vi "CANopen Read SDO.vi"() -> ()   [LabVIEW 2016]
doc: "This example demonstrates how to read CANopen SDO from the device."
uses:
  <vilib>/userdefined/High Color/nirio_resource_hc.ctl
  <vilib>/FPGAPlugInAG/cRIO-9033/niLvFpga_Open_cRIO-9033.vi
  <vilib>/rvi/interface/common/dynamic/niFpgaDynamicAddResources.vi
  <vilib>/CANopenLib/CANOPEN.llb/CANopen Interface Create.vi
  <vilib>/CANopenLib/CANOPEN.llb/CANopen SDO Create.vi
  <vilib>/CANopenLib/CANOPEN.llb/CANopen SDO Read [STR].vi
  <vilib>/CANopenLib/CANOPEN.llb/CANopen SDO Close.vi
  <vilib>/CANopenLib/CANOPEN.llb/CANopen Interface Close.vi
  <vilib>/FPGAPlugInAG/Dynamic/niLvFpga_Close_Dynamic.vi
  <vilib>/rvi/interface/nirviOpenFPGA/nirviOpenFPGA.xnode
  Users/s163601/Desktop/05-28/FPGA Bitfiles/project_FPGATarget_MainFPGA_S9ZLErdeBuw.lvbitx
  Users/s163601/Desktop/05-28/RT/FPGA/MainFPGA.vi
  <vilib>/rvi/interface/nirviCloseFPGA/nirviCloseFPGA.xnode
panel:
  out "description":string
  in  "error in":errorcluster
  out "manufacturer device name":string
  out "completion code":u32 format="%.0x"
  in  "sub-index":u8 format="%.0x"
  in  "object index":u16=4104 format="%.0x"
  in  "node-ID":u8=1 min=1 max=127 step=1
  in  "baud rate":u32(ring)=2 items=["1 Mbit/s"=0, "800 kbit/s"=1, "500 kbit/s"=2, "250 kbit/s"=3, "125 kbit/s"=4, "50 kbit/s"=6, "20 kbit/s"=7, "10 kbit/s"=8]
  in  "CANopen interface":u32(ring) items=["CANopen01", "CANopen02", "CANopen03", "CANopen04", "CANopen05", "CANopen06", "CANopen07", "CANopen08", "CANopen09", "CANopen10", "CANopen11", "CANopen12", "CANopen13", "CANopen14", "CANopen15", "CANopen16", "CANopen17", "CANopen18", "CANopen19", "CANopen20", "CANopen21", "CANopen22", "CANopen23", "CANopen24", "CANopen25", "CANopen26", "CANopen27", "CANopen28", "CANopen29", "CANopen30", "CANopen31", "CANopen32"]
  # "Overview: This example demonstrates how to read CANopen SDO from the device.\nRequirements: Connect CANopen module with a slave device. \nInstructions:\n1. Specify the values of CANopen interface, baud rate of the CANopen interface and node-ID of the slave device.\n2. Run this VI."
  # "Create CANopen interface and SDO object"
  # "Read SDO data"
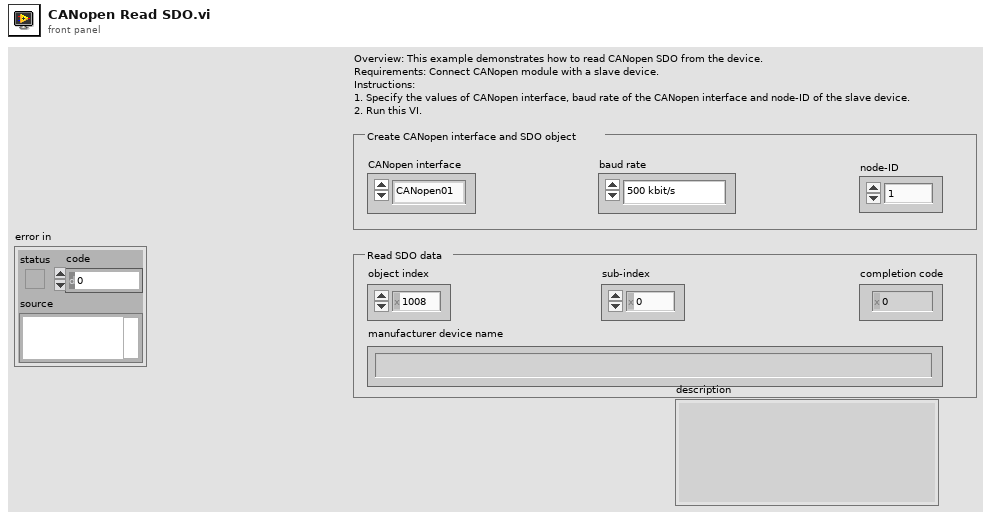
[diagram p1: front panel]
types:
  T1 = typedef "nirio_resource_hc.ctl" = tag
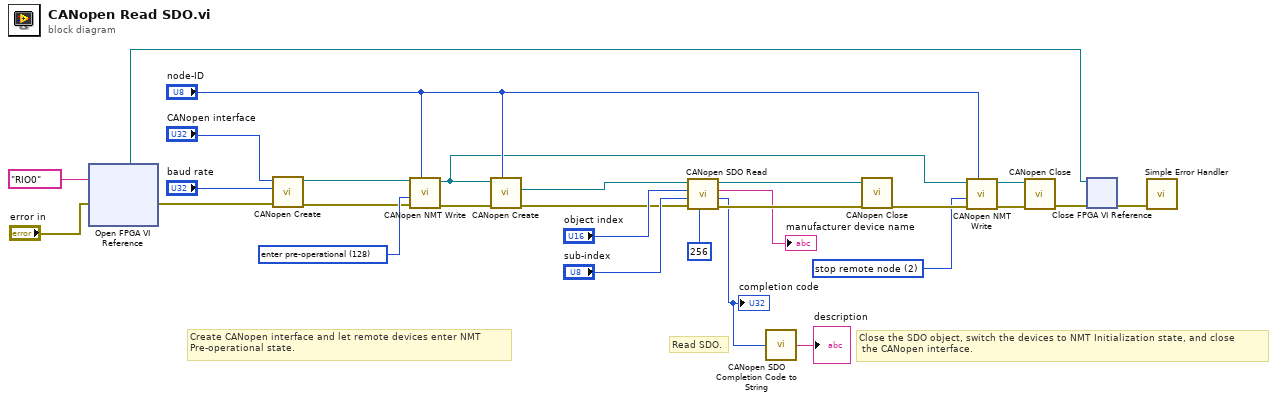
[diagram p0: block diagram]
diagram:
  w17 = u16 2 items=["start remote node"=1, "stop remote node"=2, "enter pre-operational"=128, "reset node"=129, "reset communication"=130] ("command")
  w25 = u16 128 items=["start remote node"=1, "stop remote node"=2, "enter pre-operational"=128, "reset node"=129, "reset communication"=130] ("command")
  # "Close the SDO object, switch the devices to NMT Initialization state, and close\n the CANopen interface."
  # "Create CANopen interface and let remote devices enter NMT\nPre-operational state."
  # "Read SDO."
  n1 = xnode ("Open FPGA VI Reference")("error in"="error in", "resource name"=T1 "RIO0") -> ("FPGA VI Reference Out"=w3:refnum<k20>, "error out"=w6:errorcluster)
  n2 = call-poly <vilib>:"CANopen Create.vi"("error in (no error)"=w6, "baud rate"="baud rate", "interface name"="CANopen interface") -> ("error out"=w10:errorcluster, "interface object out"=w24:refnum<k20>)  [unwired: 7 in]
  n3 = call <vilib>:"CANopen NMT Write.vi"("node-ID (0)"="node-ID", "error in (no error)"=w10, "command"=w25, "interface object in"=w24) -> ("error out"=w28:errorcluster, "interface object out"=w9:refnum<k20>)  [unwired: 6 in]
  n4 = call-poly <vilib>:"CANopen Create.vi"("node-ID"="node-ID", "error in (no error)"=w28, "interface object in"=w9) -> ("error out"=w12:errorcluster, "SDO object out"=w11:refnum<k20>)  [unwired: 6 in, 1 out]
  n5 = call-poly <vilib>:"CANopen SDO Read.vi"("data size"=u32 256, "error in (no error)"=w12, "object sub-index (0)"="sub-index", "object index"="object index", "SDO object in"=w11) -> ("error out"=w23:errorcluster, "completion code"=w2:u32, "string data"=→"manufacturer device name":string, "SDO object out"=w22:refnum<k20>)  [unwired: 3 in]
  "completion code" <- w2
  n6 = call <vilib>:"CANopen SDO Completion Code to String.vi"("SDO completion code"=w2) -> ("description"=→"description":string)
  n7 = call-poly <vilib>:"CANopen Close.vi"("error in (no error)"=w23, "SDO object in"=w22) -> ("error out"=w19:errorcluster)  [unwired: 9 in]
  n8 = call <vilib>:"CANopen NMT Write.vi"("node-ID (0)"="node-ID", "error in (no error)"=w19, "command"=w17, "interface object in"=w9) -> ("error out"=w16:errorcluster, "interface object out"=w15:refnum<k20>)  [unwired: 6 in]
  n9 = call-poly <vilib>:"CANopen Close.vi"("error in (no error)"=w16, "interface object in"=w15) -> ("error out"=w5:errorcluster)  [unwired: 9 in]
  n10 = xnode "Close FPGA VI Reference"("FPGA VI Reference In"=w3, "error in"=w5) -> ("error out"=w4:errorcluster)
  n11 = call <vilib>:"Simple Error Handler.vi"("error in (no error)"=w4) -> ()  [unwired: 4 in, 5 out]
